vi "_script_fix_Parse State Queue in Find Parse State Queue vi name2.vi"   [LabVIEW 2014]
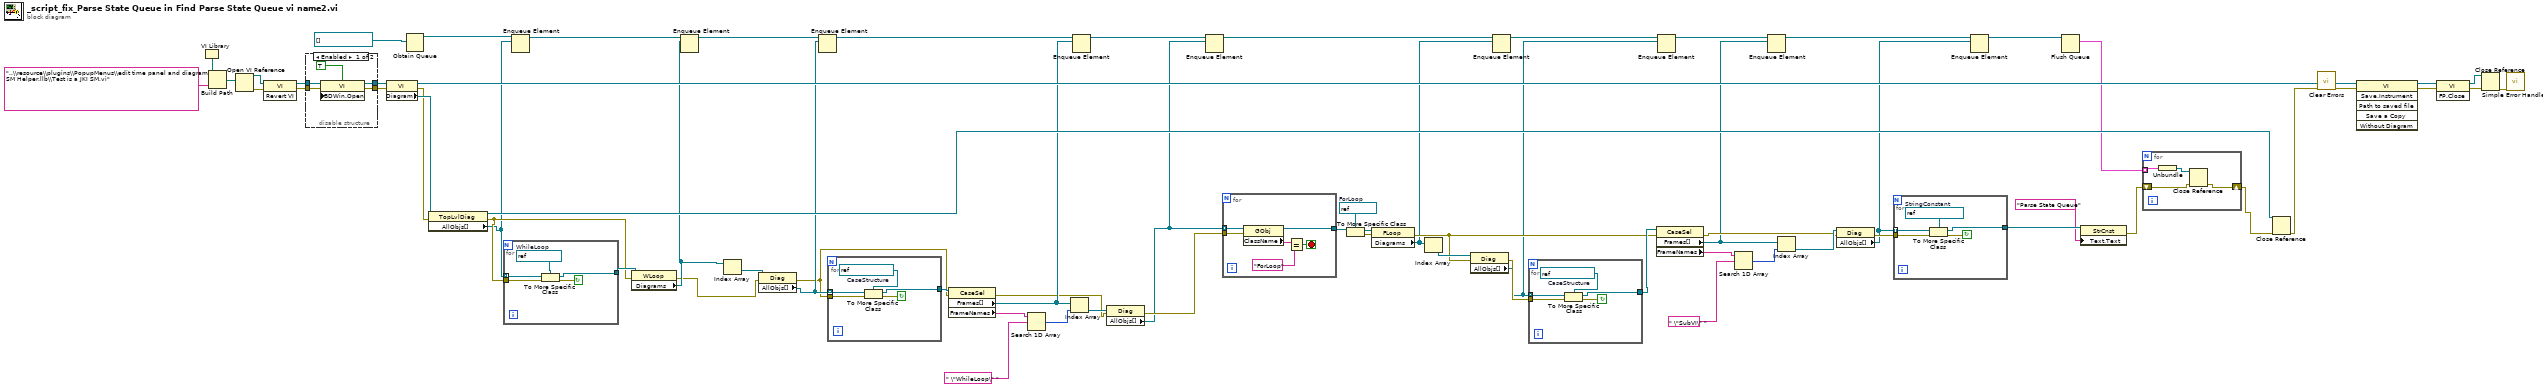
[diagram p0: block diagram]
diagram:
  w61 = refnum<vi> refnum  # ForLoop
  n1 = VI Library() -> (path=w69:path)
  n2 = Build Path(base path=w69, name or relative path="..\\resource\\plugins\\PopupMenus\\edit time panel and diagram\\JKI SM Helper.llb\\Test is a JKI SM.vi") -> (appended path=w67:path)
  n3 = Open VI Reference(vi path=w67) -> (vi reference=w70:refnum<vi>, error out=w71:errorcluster)  [unwired: 5 in]
  n4 = invoke class="VI" method="Revert VI"(reference=w70, error in=w71) -> (reference out=w53:refnum<vi>, error out=w52:errorcluster)  [unwired: 1 in, 1 out]
  n5 = disable-structure shown="Enabled" {
    disable-tunnel: w53 -> [w76 w78]
    disable-tunnel: w52 -> [w75 w77]
    disable-tunnel: [w74 w78] -> w51
    disable-tunnel: [w73 w77] -> w50
    frame Enabled {
      n6 = property class="VI"(reference=w76, error in=w75, "BDWin.Open"=TRUE ("Block Diagram Window:Open")) -> (reference out=w74:refnum<vi>, error out=w73:errorcluster)
    }
    frame Disabled {
    }
  }
  n7 = property class="VI"(reference=w51, error in=w50) -> (reference out=w66:refnum<vi>, error out=w63:errorcluster, "Diagram"=w64:refnum<vi>)
  n8 = Obtain Queue(element data type=refnum<vi>[] [] ("All Objects[]")) -> (queue out=w37:refnum<queue>)  [unwired: 4 in, 2 out]
  n9 = property class="TopLvlDiag"(reference=w64, error in=w63) -> (reference out=w55:refnum<vi>, error out=w39:errorcluster, "AllObjs[]"=w36:refnum<vi>[])
  n10 = for {
    tunnel: w36 -> [w83] mode=indexing
    tunnel: w39 -> [w82]
    tunnel: [w80] -> w40
    stop <- w81 continue-if-true
    w79 = refnum<vi> refnum  # WhileLoop
    n11 = To More Specific Class(target class=w79, reference=w83, error in=w82) -> (specific class reference=w80:refnum<vi>, error out=w81:errorcluster)
  }
  n12 = Enqueue Element(queue=w37, element=w36) -> (queue out=w35:refnum<queue>)  [unwired: 2 in, 2 out]
  n13 = property class="WLoop"(reference=w40, error in=w39) -> (error out=w32:errorcluster, "Diagrams"=w34:refnum<vi>[])  [unwired: 1 out]
  n14 = Enqueue Element(queue=w35, element=w34) -> (queue out=w30:refnum<queue>)  [unwired: 2 in, 2 out]
  n15 = Index Array(array=w34) -> (element=w33:refnum<vi>)  [unwired: 1 in]
  n16 = property class="Diag"(reference=w33, error in=w32) -> (error out=w23:errorcluster, "AllObjs[]"=w31:refnum<vi>[])  [unwired: 1 out]
  n17 = Enqueue Element(queue=w30, element=w31) -> (queue out=w25:refnum<queue>)  [unwired: 2 in, 2 out]
  n18 = for {
    tunnel: w31 -> [w88] mode=indexing
    tunnel: w23 -> [w87]
    tunnel: [w85] -> w26
    stop <- w86 continue-if-true
    w84 = refnum<vi> refnum  # CaseStructure
    n19 = To More Specific Class(target class=w84, reference=w88, error in=w87) -> (specific class reference=w85:refnum<vi>, error out=w86:errorcluster)
  }
  n20 = property class="CaseSel"(reference=w26, error in=w23) -> (error out=w21:errorcluster, "Frames[]"=w24:refnum<vi>[], "FrameNames"=w27:string[])  [unwired: 1 out]
  n21 = Search 1D Array(1D array=w27, element=" \"WhileLoop\" " ("y")) -> (index of element=w29:i32)  [unwired: 1 in]
  n22 = Index Array(array=w24, index=w29) -> (element=w22:refnum<vi>)
  n23 = Enqueue Element(queue=w25, element=w24) -> (queue out=w18:refnum<queue>)  [unwired: 2 in, 2 out]
  n24 = property class="Diag"(reference=w22, error in=w21) -> (error out=w20:errorcluster, "AllObjs[]"=w19:refnum<vi>[])  [unwired: 1 out]
  n25 = Enqueue Element(queue=w18, element=w19) -> (queue out=w16:refnum<queue>)  [unwired: 2 in, 2 out]
  n26 = for {
    tunnel: w19 -> [w94] mode=indexing
    tunnel: w20 -> [w93]
    tunnel: [w92] -> w62
    stop <- w89 stop-if-true
    n27 = property class="GObj"(reference=w94, error in=w93) -> (reference out=w92:refnum<vi>, "ClassName"=w91:string)  [unwired: 1 out]
    n28 = Equal?(x=w91, y="ForLoop") -> (x = y?=w89:bool)
  }
  n29 = To More Specific Class(target class=w61, reference=w62) -> (specific class reference=w60:refnum<vi>, error out=w59:errorcluster)  [unwired: 1 in]
  n30 = property class="FLoop"(reference=w60, error in=w59) -> (error out=w46:errorcluster, "Diagrams"=w17:refnum<vi>[])  [unwired: 1 out]
  n31 = Index Array(array=w17) -> (element=w49:refnum<vi>)  [unwired: 1 in]
  n32 = property class="Diag"(reference=w49, error in=w46) -> (error out=w48:errorcluster, "AllObjs[]"=w14:refnum<vi>[])  [unwired: 1 out]
  n33 = Enqueue Element(queue=w16, element=w17) -> (queue out=w15:refnum<queue>)  [unwired: 2 in, 2 out]
  n34 = for {
    tunnel: w14 -> [w99] mode=indexing
    tunnel: w48 -> [w98]
    tunnel: [w96] -> w47
    stop <- w97 continue-if-true
    w95 = refnum<vi> refnum  # CaseStructure
    n35 = To More Specific Class(target class=w95, reference=w99, error in=w98) -> (specific class reference=w96:refnum<vi>, error out=w97:errorcluster)
  }
  n36 = property class="CaseSel"(reference=w47, error in=w46) -> (error out=w41:errorcluster, "Frames[]"=w13:refnum<vi>[], "FrameNames"=w45:string[])  [unwired: 1 out]
  n37 = Enqueue Element(queue=w15, element=w14) -> (queue out=w12:refnum<queue>)  [unwired: 2 in, 2 out]
  n38 = Search 1D Array(1D array=w45, element=" \"SubVI\" " ("y")) -> (index of element=w43:i32)  [unwired: 1 in]
  n39 = Enqueue Element(queue=w12, element=w13) -> (queue out=w11:refnum<queue>)  [unwired: 2 in, 2 out]
  n40 = Index Array(array=w13, index=w43) -> (element=w42:refnum<vi>)
  n41 = property class="Diag"(reference=w42, error in=w41) -> (error out=w58:errorcluster, "AllObjs[]"=w10:refnum<vi>[])  [unwired: 1 out]
  n42 = for {
    tunnel: w10 -> [w104] mode=indexing
    tunnel: w58 -> [w103]
    tunnel: [w100] -> w57
    stop <- w101 continue-if-true
    w102 = refnum<vi> refnum  # StringConstant
    n43 = To More Specific Class(target class=w102, reference=w104, error in=w103) -> (specific class reference=w100:refnum<vi>, error out=w101:errorcluster)
  }
  n44 = Enqueue Element(queue=w11, element=w10) -> (queue out=w9:refnum<queue>)  [unwired: 2 in, 2 out]
  n45 = Flush Queue(queue=w9) -> (remaining elements=w8:cluster{"All Objects[]":refnum<vi>[]}[])  [unwired: 1 in, 2 out]
  n46 = property class="StrCnst"(reference=w57, "Text.Text"="Parse State Queue") -> (error out=w7:errorcluster)  [unwired: 1 in, 1 out]
  n47 = for {
    tunnel: w8 -> [w108] mode=indexing
    shift-right: [w105] -> w6
    shift-left: w7 -> [w106]
    n48 = Unbundle(w108) -> ("All Objects[]"=w107:refnum<vi>[])
    n49 = Close Reference(reference=w107, error in (no error)=w106) -> (error out=w105:errorcluster)
  }
  n50 = Close Reference(reference=w55, error in (no error)=w6) -> (error out=w54:errorcluster)
  n51 = call <vilib>:"Clear Errors.vi"("error in (no error)"=w54) -> ("error out"=w1:errorcluster)  [unwired: 6 in]
  n52 = invoke class="VI" method="Save.Instrument"(reference=w66, error in=w1) -> (reference out=w4:refnum<vi>, error out=w5:errorcluster)  [unwired: 4 in, 4 out]
  n53 = invoke class="VI" method="FP.Close"(reference=w4, error in=w5) -> (reference out=w2:refnum<vi>, error out=w3:errorcluster)  [unwired: 1 in, 1 out]
  n54 = Close Reference(reference=w2, error in (no error)=w3) -> (error out=w65:errorcluster)
  n55 = call <vilib>:"Simple Error Handler.vi"("error in (no error)"=w65) -> ()  [unwired: 4 in, 5 out]
